vi "HDMIDiffractiveTest.vi"() -> ()   [LabVIEW 2010]
uses:
  Program Files/Meadowlark Optics/Blink 1920 HDMI/SDK/Blink_C_wrapper.dll
  <vilib>/Utility/file.llb/Write To Spreadsheet File (I64).vi
  ImageGen.dll
panel:
  out "Array":u8[][](array[numeric])
  # "Load diffraction patterns to the SLM, and measure 1st order intensity to calibrate a LUT\nCan be used to generate a global or regional LUT"
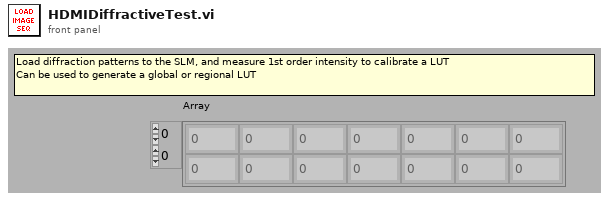
[diagram p1: front panel]
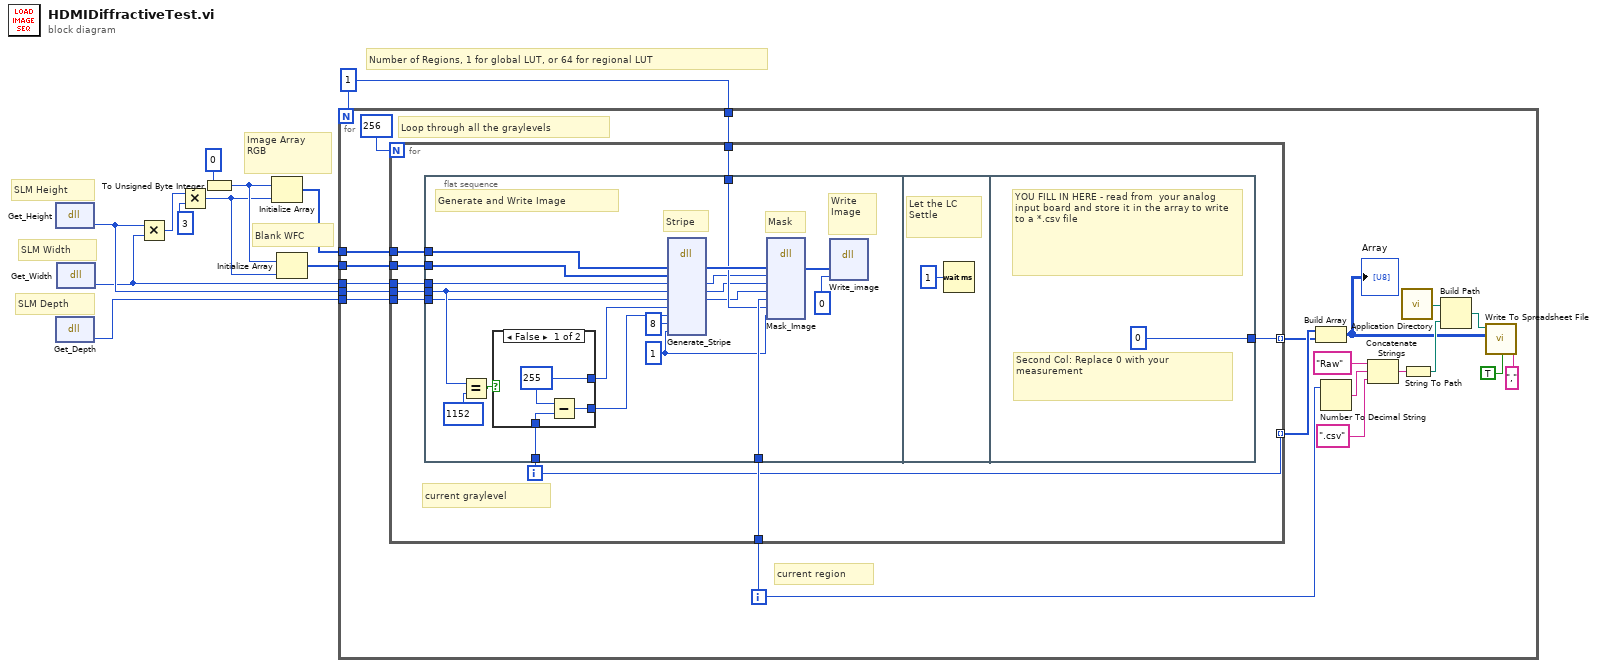
[diagram p0: block diagram]
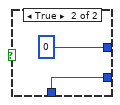
[diagram p2: hidden frame]
diagram:
  w9 = 1
  # "Blank WFC"
  # "SLM Depth"
  # "Number of Regions, 1 for global LUT, or 64 for regional LUT"
  # "SLM Width"
  # "SLM Height"
  # "Image Array\nRGB"
  n1 = dll-call lib="C:/Program Files/Meadowlark Optics/Blink 1920 HDMI/SDK/Blink_C_wrapper.dll" fn="Get_Height"() -> ("return type"=w8:i32)  [unwired: 3 in, 2 out]
  n2 = dll-call lib="C:/Program Files/Meadowlark Optics/Blink 1920 HDMI/SDK/Blink_C_wrapper.dll" fn="Get_Depth"() -> ("return type"=w1:i32)  [unwired: 3 in, 2 out]
  n3 = dll-call lib="C:/Program Files/Meadowlark Optics/Blink 1920 HDMI/SDK/Blink_C_wrapper.dll" fn="Get_Width"() -> ("return type"=w7:i32)  [unwired: 3 in, 2 out]
  n4 = Multiply(x=w8, y=w7) -> (x*y=w6:i32)
  n5 = Multiply(x=w6, y=3) -> (x*y=w3:i32)
  n6 = To Unsigned Byte Integer(number=0) -> (unsigned 8bit integer=w4:u8)
  n7 = Initialize Array(w4, w3) -> (w10:u8[])
  n8 = Initialize Array(w4, w3) -> (w2:u8[])
  n9 = for {
    N: w9 -> [_]
    tunnel: w10 -> [w31]
    tunnel: w7 -> [w30]
    tunnel: w8 -> [w29]
    tunnel: w9 -> [w27]
    tunnel: w2 -> [w13]
    tunnel: w1 -> [w12]
    i -> [w25]
    # "Loop through all the graylevels"
    # "current region"
    n10 = for {
      N: 256 -> [_]
      tunnel: w31 -> [w40]
      tunnel: w30 -> [w39]
      tunnel: w29 -> [w38]
      tunnel: w25 -> [w37]
      tunnel: w27 -> [w36]
      tunnel: [w35] -> w15 mode=indexing
      tunnel: [w34] -> w14 mode=indexing
      tunnel: w13 -> [w33]
      tunnel: w12 -> [w32]
      i -> [w35]
      # "current graylevel"
      n11 = flat-sequence {
        tunnel: w40 -> [w60]
        tunnel: w39 -> [w58]
        tunnel: w38 -> [w52]
        tunnel: w37 -> [w55]
        tunnel: w36 -> [w54]
        tunnel: w35 -> [w49]
        tunnel: w33 -> [w46]
        tunnel: w32 -> [w45]
        tunnel: [0] -> w34
        frame #0 {
          w41 = 1
          # "Generate and Write Image"
          # "Write \nImage"
          # "Mask"
          # "Stripe"
          n12 = Equal?(x=w52, y=1152) -> (x = y?=w50:bool)
          n13 = case shown="False" w50 {
            tunnel: w49 -> [w63 w64]
            tunnel: [w62 0] -> w48
            tunnel: [w61 w64] -> w47
            frame False {
              w62 = 255
              n14 = Subtract(x=w62, y=w63) -> (x-y=w61:i32)
            }
            frame True {
            }
          }
          n15 = dll-call lib="C:/Meadowlark/Repos-git/MeadowlarkBison/BlinkSdkExample/ImageGen.dll" fn="Generate_Stripe"("Array"=w60, "WFC"=w46, "Width"=w58, "Height"=w52, "Depth"=w45, "PixelValOne"=w48, "PixelValTwo"=w47, "PixelsPerStripe"=8, "RGB"=w41) -> ("Array"=w59:u8[], "Width"=w42:i32, "Height"=w43:i32, "Depth"=w44:i32)  [unwired: 9 in, 2 out]
          n16 = dll-call lib="C:/Meadowlark/Repos-git/MeadowlarkBison/BlinkSdkExample/ImageGen.dll" fn="Mask_Image"("Array"=w59, "Width"=w42, "Height"=w43, "Depth"=w44, "Region"=w55, "NumRegions"=w54, "RGB"=w41) -> ("Array"=w56:u8[])  [unwired: 10 in, 2 out]
          n17 = dll-call lib="C:/Program Files/Meadowlark Optics/Blink 1920 HDMI/SDK/Blink_C_wrapper.dll" fn="Write_image"("image_data"=w56, "isEightBit"=0) -> ()  [unwired: 6 in, 2 out]
        }
        frame #1 {
          # "Let the LC \nSettle"
          n18 = Wait (ms)(milliseconds to wait=u32 1) -> ()  [unwired: 1 out]
        }
        frame #2 {
          # "Second Col: Replace 0 with your measurement"
          # "YOU FILL IN HERE - read from  your analog input board and store it in the array to write to a *.csv file"
        }
      }
    }
    n19 = Build Array(w15, w14) -> (w16:i32[][])
    "Array" <- w16
    n20 = Number To Decimal String(number=w25) -> (decimal integer string=w24:string)  [unwired: 1 in]
    n21 = Concatenate Strings("Raw", w24, ".csv") -> (w22:string)
    n22 = call <vilib>:"Application Directory.vi"() -> ("Application Directory"=w21:path)
    n23 = String To Path(string=w22) -> (path=w20:path)
    n24 = Build Path(base path=w21, name or relative path=w20) -> (appended path=w19:path)
    n25 = call-poly <vilib>:"Write To Spreadsheet File.vi"("delimiter (\\t)"=",", "transpose? (no:F)"=TRUE, "2D data"=w16, "file path (dialog if empty)"=w19) -> ()  [unwired: 4 in, 1 out]
  }
